vi "agilent_temps_backup.vi"(6 "error in (no error)":errorcluster, 10 "Readings":u16=1, 11 "Agilent Port In":refnum<visa-resource-name>="COM35") -> (0 "Room T":dbl=22.39480077719182, 1 "Brt T":dbl=22.603658046093727, 2 "Acid T":dbl=20.114285856024708, 3 "Cell T":dbl=20.11450810063397, 4 "error out":errorcluster, 5 "Agilent Port Out":refnum<visa-resource-name>="COM35")   [LabVIEW 2010]
uses:
  ProbeClass/TempProbeSet.lvclass
panel:
  in  "TempProbeSet in":refnum<class "TempProbeSet.lvclass">
  # "mooseNote: takes the resistance measurements from the Agilent, looks up the calibration functions in a table and spits out scaled temperatures"
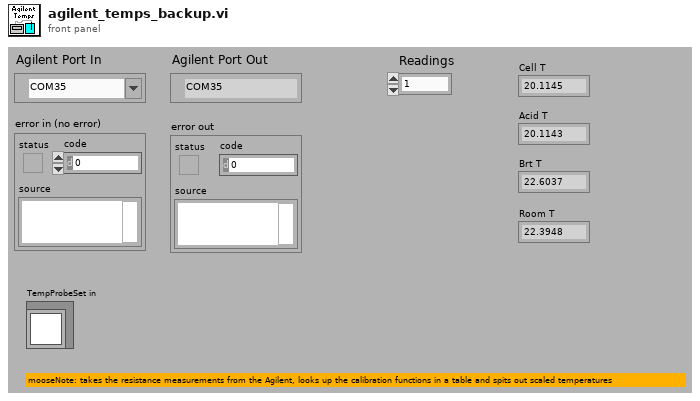
[diagram p1: front panel]
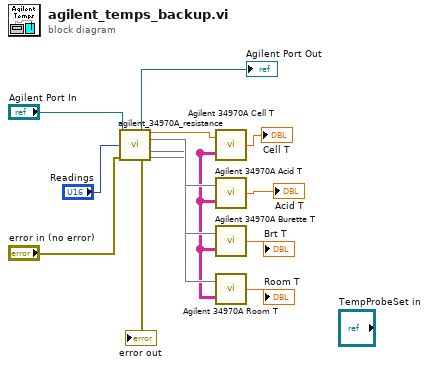
[diagram p0: block diagram]
diagram:
  n1 = call "agilent_34970A_resistance.vi"("Agilent Port In"="Agilent Port In", "Readings"="Readings", "error in (no error)"="error in (no error)") -> ("Agilent Port Out"=→"Agilent Port Out":refnum<visa-resource-name>, "Avg R1"=w12:dbl, 6:w9, 10:w8, "error out"=→"error out":errorcluster, 15:w6)  [unwired: 6 in, 1 out]
  n2 = call "Agilent 34970A Burette T.vi"("Resistance"=w8) -> ("Brt T"=→"Brt T":dbl, "Therm Coefs"=w4:string[][])
  n3 = call "Agilent 34970A Cell T.vi"("Therm Coefs"=w4, "Resistance"=w12) -> ("Cell T"=→"Cell T":dbl)
  n4 = call "Agilent 34970A Acid T.vi"("Therm Coefs"=w4, "Resistance"=w9) -> ("Acid T"=→"Acid T":dbl)
  n5 = call "Agilent 34970A Room T.vi"("Therm Coefs"=w4, "Resistance"=w6) -> ("Room T"=→"Room T":dbl)
